vi "putMine.vi"(8 "error in (no error)":errorcluster, 11 "Cell in":refnum<class "Cell.lvclass">) -> (0 "error out":errorcluster, 3 "Cell out":refnum<class "Cell.lvclass">)   [LabVIEW 2014, in "Cell.lvclass"]
uses:
  Cell.lvclass
  Cell.lvclass/Cell.ctl
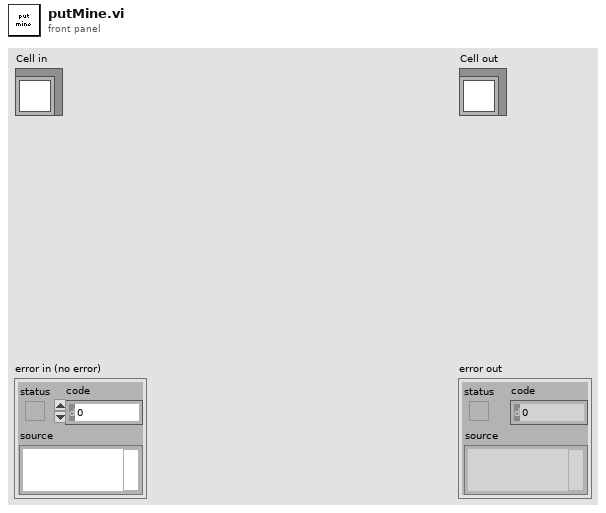
[diagram p1: front panel]
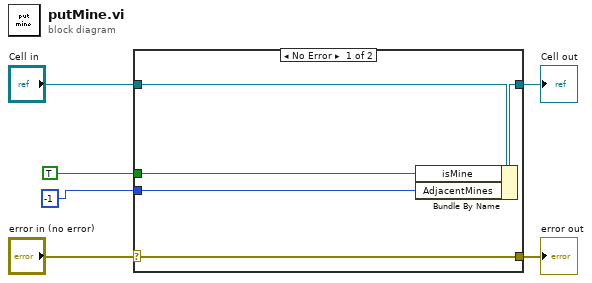
[diagram p0: block diagram]
diagram:
  n1 = case shown="No Error" "error in (no error)" {
    selector: "error in (no error)" -> [w11 w12]
    tunnel: [w11 w12] -> w5
    tunnel: [w9 w13] -> w3
    tunnel: "Cell in" -> [w10 w13]
    tunnel: TRUE ("isMine") -> [w8 _]
    tunnel: -1 -> [w7 _]
    frame No Error {
      n2 = Bundle By Name(cluster=w10, "isMine"=w8, "AdjacentMines"=w7) -> (w9:refnum<class "Cell.lvclass">)
    }
    frame Error {
    }
  }
  "error out" <- w5
  "Cell out" <- w3
